vi "rad_Apply Network Settings (Static).vi"(5 "Password":string, 8 "error in (no error)":errorcluster, 10 "Requested settings":T1={"Hostname"="", "Serial number"="", "Product name"="", "Product code"=0, "System status"="", "Credential type"=enum."None/Unlocked", "User added?"=FALSE, "Primary NIC"={"MAC address"="", "IP Address Request Mode"=2, "IP address"="", "Subnet mask"="", "Gateway"="", "DNS server"=""}} {"Primary NIC"."IP Address Request Mode" items=["Static"=1, "DHCP/Link-Local"=2, "Link-Local Only"=4, "DHCP Only"=8]}, 11 "Existing settings":T1={"Hostname"="", "Serial number"="", "Product name"="", "Product code"=0, "System status"="", "Credential type"=enum."None/Unlocked", "User added?"=FALSE, "Primary NIC"={"MAC address"="", "IP Address Request Mode"=2, "IP address"="", "Subnet mask"="", "Gateway"="", "DNS server"=""}} {"Primary NIC"."IP Address Request Mode" items=["Static"=1, "DHCP/Link-Local"=2, "Link-Local Only"=4, "DHCP Only"=8]}) -> (0 "error out":errorcluster, 3 "Target settings out":T1={"Hostname"="", "Serial number"="", "Product name"="", "Product code"=0, "System status"="", "Credential type"=enum."None/Unlocked", "User added?"=FALSE, "Primary NIC"={"MAC address"="", "IP Address Request Mode"=2, "IP address"="", "Subnet mask"="", "Gateway"="", "DNS server"=""}} {"Primary NIC"."IP Address Request Mode" items=["Static"=1, "DHCP/Link-Local"=2, "Link-Local Only"=4, "DHCP Only"=8]})   [LabVIEW 2020]
uses:
  <resource>/objmgr/nisysapi.rc
  <vilib>/nisyscfg/nisyscfg.lvlib
  <vilib>/nisyscfg/Save Changes (System).vi
  <vilib>/nisyscfg/Close (System).vi
  rad_Globals.vi
  TypeDefs/rad_Target Information.ctl
  TypeDefs/rad_Target Network Settings.ctl
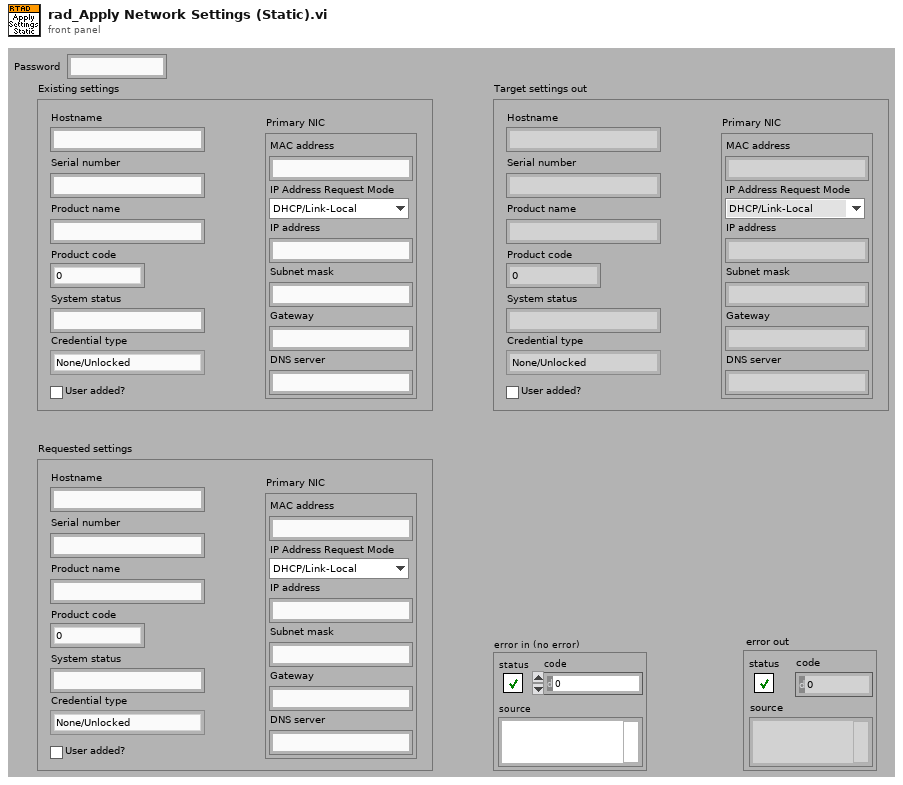
[diagram p1: front panel]
types:
  T1 = typedef "rad_Target Information.ctl" = cluster{"Hostname":string, "Serial number":string, "Product name":string, "Product code":i32, "System status":string, "Credential type":enum16{"None/Unlocked", "FTP Password", "NIAuth Credentials"}, "User added?":bool, "Primary NIC":T2}
  T2 = typedef "rad_Target Network Settings.ctl" = cluster{"MAC address":string, "IP Address Request Mode":i32, "IP address":string, "Subnet mask":string, "Gateway":string, "DNS server":string}
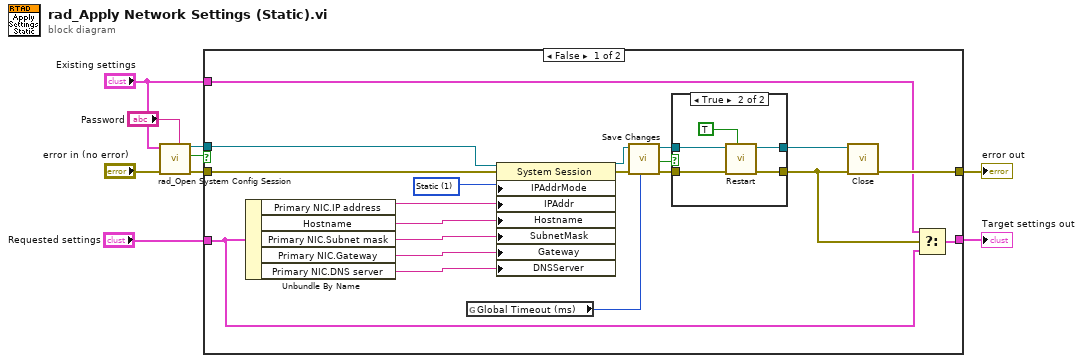
[diagram p0: block diagram]
diagram:
  n1 = call "rad_Open System Config Session.vi"("Password"="Password", "error in (no error)"="error in (no error)", "Target settings"="Existing settings") -> ("error out"=w6:errorcluster, "Cancelled"=w5:bool, "Session out"=w7:refnum<k21>)  [unwired: 5 in, 1 out]
  n2 = case shown="False" w5 {
    tunnel: [w11 w37] -> w2
    tunnel: [w29 w38] -> w8
    tunnel: w7 -> [w28 _]
    tunnel: "Requested settings" -> [w12 _]
    tunnel: w6 -> [w15 w38]
    tunnel: "Existing settings" -> [w13 w37]
    frame False {
      w22 = 1 items=["Static"=1, "DHCP/Link-Local"=2, "Link-Local Only"=4, "DHCP Only"=8] ("Primary NIC:IP Address Request Mode")
      n3 = Unbundle By Name(w12) -> ("Primary NIC.IP address"=w27:string, "Hostname"=w26:string, "Primary NIC.Subnet mask"=w25:string, "Primary NIC.Gateway"=w24:string, "Primary NIC.DNS server"=w23:string)
      n4 = global read "rad_Globals.vi" "Global Timeout (ms)"() -> (w10:u32)
      n5 = property class="System Session"(reference=w28, error in=w15, "IPAddrMode"=w22, "IPAddr"=w27, "Hostname"=w26, "SubnetMask"=w25, "Gateway"=w24, "DNSServer"=w23) -> (reference out=w21:refnum<k21>, error out=w20:errorcluster)
      n6 = call-poly <vilib>:"Save Changes.vi"("Remote Timeout (300,000 ms)"=w10, "error in (no error)"=w20, "Session in"=w21) -> ("error out"=w18:errorcluster, "Changes Require Restart"=w19:bool, "Session out"=w17:refnum<k21>)  [unwired: 5 in, 1 out]
      n7 = case shown="True" w19 {
        tunnel: w18 -> [w31 w36]
        tunnel: [w31 w35] -> w14
        tunnel: w17 -> [w30 w34]
        tunnel: [w30 w33] -> w16
        frame False {
        }
        frame True {
          n8 = call <vilib>:"Restart.vi"("Wait Until Complete (T)"=TRUE ("wait until complete (T)"), "error in (no error)"=w36, "Session in"=w34) -> ("error out"=w35:errorcluster, "Session out"=w33:refnum<k21>)  [unwired: 6 in, 1 out]
        }
      }
      n9 = call-poly <vilib>:"Close.vi"("error in (no error)"=w14, "Session in"=w16) -> ("error out"=w29:errorcluster)  [unwired: 9 in]
      n10 = Select(t=w13, s=w14, f=w12) -> (s? t:f=w11:T1)
    }
    frame True {
    }
  }
  "error out" <- w8
  "Target settings out" <- w2
